vi "change_string_to_action.vi"(11 "String":string) -> (2 "output cluster 2":cluster{i32, i32, i32}, 3 "output cluster":cluster{i32, i32, i32})   [LabVIEW 2025]
panel:
  in  "Array":i32[](array[numeric])
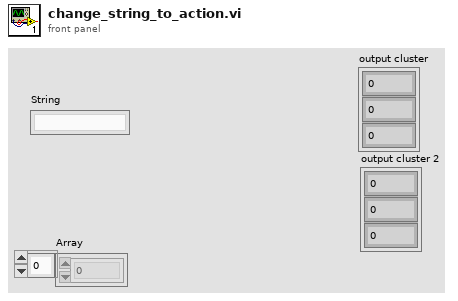
[diagram p1: front panel]
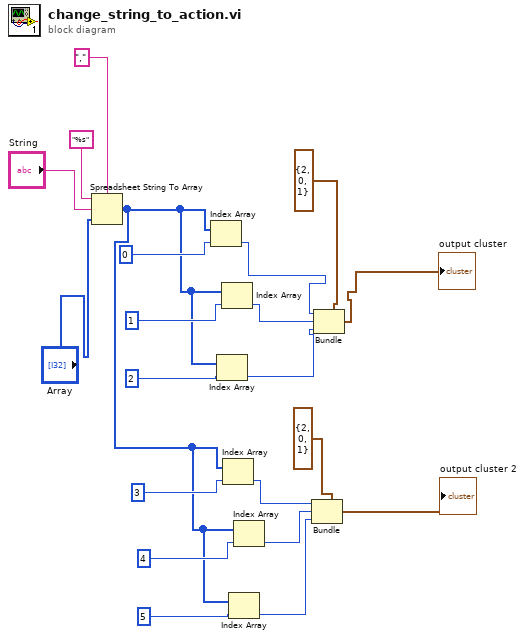
[diagram p0: block diagram]
diagram:
  n1 = Spreadsheet String To Array(delimiter (Tab)=",", format string="%s", spreadsheet string="String", array type (2D Dbl)="Array") -> (array=w3:i32[])
  n2 = Index Array(array=w3, index=0) -> (element=w15:i32)
  n3 = Index Array(array=w3, index=2) -> (element=w13:i32)
  n4 = Index Array(array=w3, index=1) -> (element=w14:i32)
  n5 = Index Array(array=w3, index=3) -> (element=w4:i32)
  n6 = Index Array(array=w3, index=5) -> (element=w1:i32)
  n7 = Index Array(array=w3, index=4) -> (element=w2:i32)
  n8 = Bundle(cluster=cluster{i32, i32, i32} {2, 0, 1} ("moves"), w4, w2, w1) -> (→"output cluster 2":cluster{i32, i32, i32})
  n9 = Bundle(cluster=cluster{i32, i32, i32} {2, 0, 1} ("moves"), w15, w14, w13) -> (→"output cluster":cluster{i32, i32, i32})
